vi "GetCycleNumber.vi"(10 "coordinate":T1, 11 "AI_Snake in":refnum<class "AI_Snake.lvclass">) -> (3 "CycleNumber":i16)   [LabVIEW 2019, in "RT_Game.lvlib" / "AI_Snake.lvclass"]
uses:
  AI_Snake.lvclass
  Engine/Coordinate.ctl
  AI_Snake.lvclass/AI_Snake.ctl
  Engine/Engine.lvclass
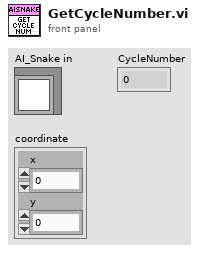
[diagram p1: front panel]
types:
  T1 = typedef "RT_Game.lvlib/Engine.lvclass/Coordinate.ctl" = cluster{"x":dbl, "y":dbl}
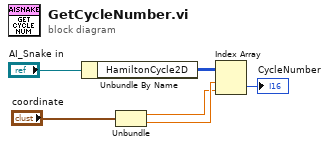
[diagram p0: block diagram]
diagram:
  n1 = Unbundle By Name("AI_Snake in") -> ("HamiltonCycle2D"=w5:i16[][])
  n2 = Unbundle("coordinate") -> ("x"=w3:dbl, "y"=w4:dbl)
  n3 = Index Array(array=w5, index (row)=w4, index (col)=w3) -> (element=→"CycleNumber":i16)
